vi "Global.vi"() -> ()   [LabVIEW 2015]
panel:
  in  "MES参数":T1
  in  "运行状态位置":i32
  out "气密保持压力持续时间":string
  out "气密充气时间":string
  out "气密保持压力":string
  out "运行状态时间点":dbl[](array[numeric])
  out "PACK编码":string
  out "员工编号":string
  out "mes抬头":string[][](array[string])
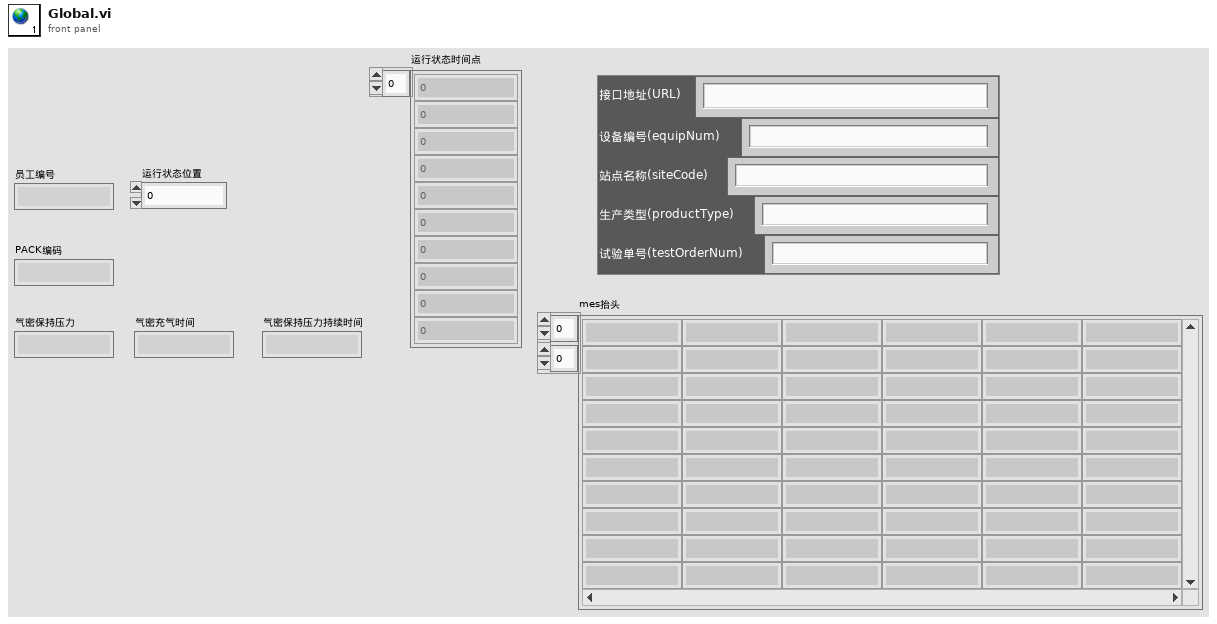
[diagram p1: front panel]
types:
  T1 = cluster{"接口地址(URL)":string, "设备编号(equipNum)":string, "站点名称(siteCode)":string, "生产类型(productType)":string, "试验单号(testOrderNum)":string}
diagram:
